vi "MV decode status.vi"(10 "status byte":i16) -> (2 "status cluster":T1)   [LabVIEW 2015, in "Millennia V.lvclass"]
doc: "Takes a status byte from the Millennia V laser and returns a cluster of booleans indicating which bits were set."
uses:
  Millennia V.lvclass
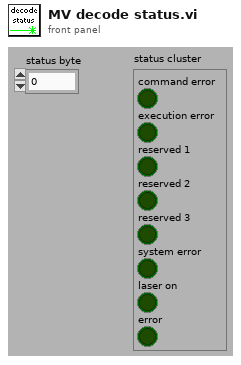
[diagram p1: front panel]
types:
  T1 = cluster{"command error":bool, "execution error":bool, "system error":bool, "laser on":bool, "error":bool, "reserved 1":bool, "reserved 2":bool, "reserved 3":bool}
  T2 = cluster{"Boolean array[0]":bool, "Boolean array[1]":bool, "Boolean array[2]":bool, "Boolean array[3]":bool, "Boolean array[4]":bool, "Boolean array[5]":bool, "Boolean array[6]":bool, "Boolean array[7]":bool}
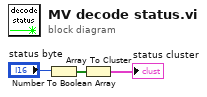
[diagram p0: block diagram]
diagram:
  n1 = Number To Boolean Array(number="status byte") -> (Boolean array=w2:bool[])
  n2 = Array To Cluster(array=w2) -> (cluster=→"status cluster":T2)
